vi "selectDailySummary.vi"(8 "Shift":string="中", 10 "End_date":string="2014/11/13", 11 "Begin_date":string="2014/11/12") -> (2 "Summary":string[][](array[string]))   [LabVIEW 2012]
uses:
  <vilib>/addons/database/Auxilliary.llb/DB Tools Cursor Type.ctl
  <vilib>/addons/database/Connection.llb/DB Tools Open Connec (Path).vi
  <vilib>/addons/database/Connection.llb/Conn Execute.vi
  <vilib>/addons/database/Recordset.llb/Rec Fetch Recordset Data (R).vi
  <vilib>/addons/database/Recordset.llb/Rec Destroy - Connection.vi
  <vilib>/addons/database/_DB Variant To Data/Database Variant To Data.xnode
  <vilib>/addons/database/NI_Database_API.lvlib
panel:
  out "concatenated string":string
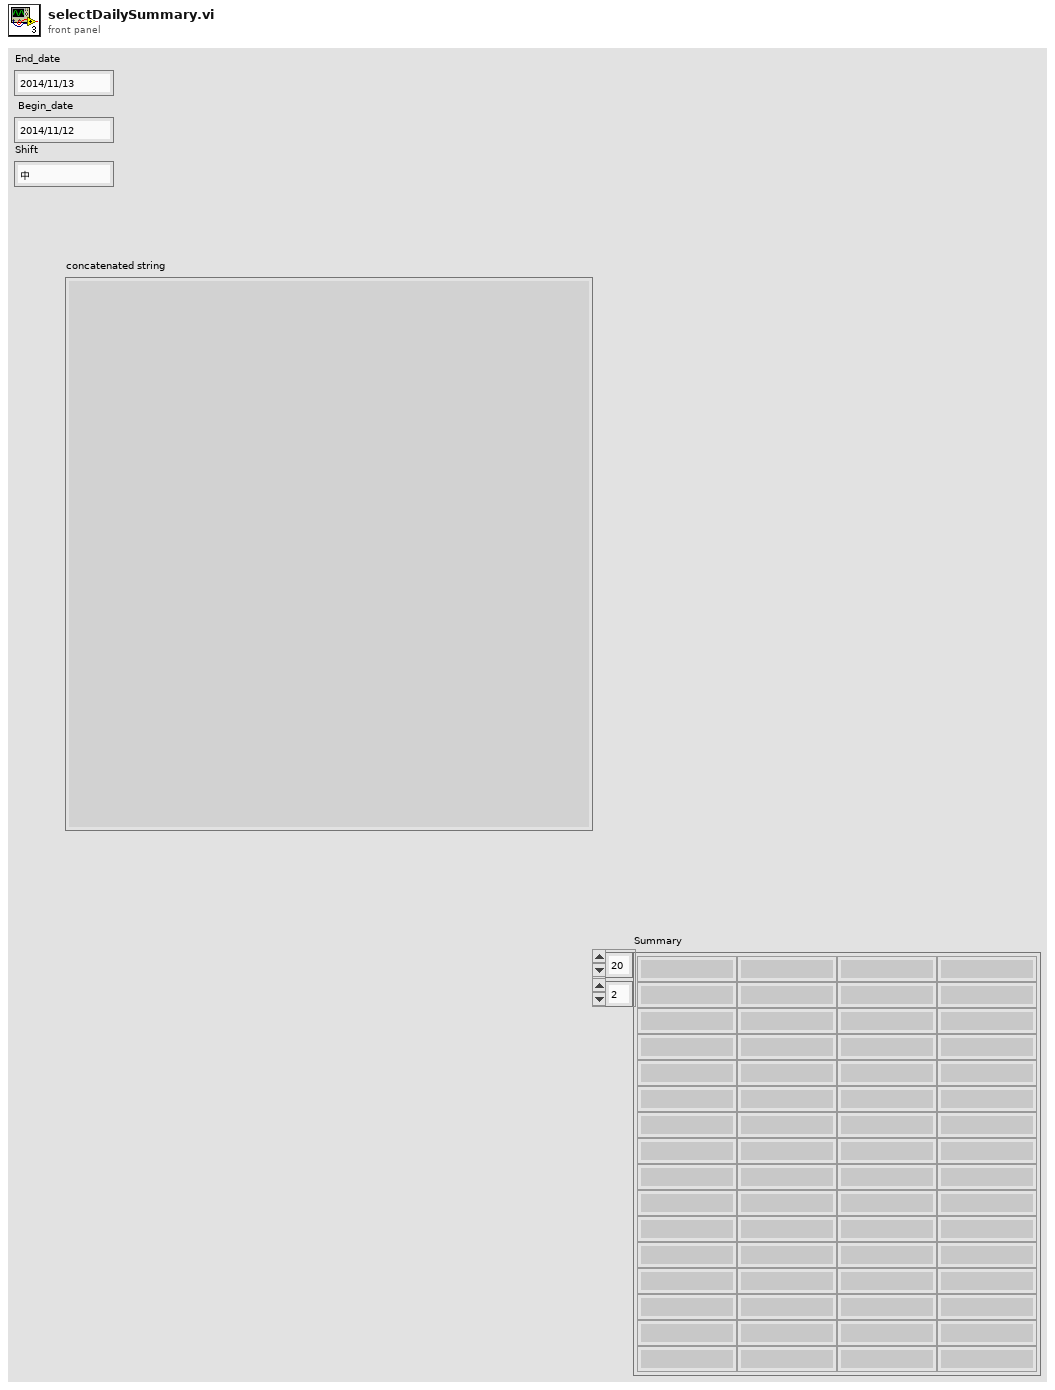
[diagram p1: front panel]
types:
  T1 = typedef "NI_Database_API.lvlib/DB Tools Cursor Type.ctl" = enum16{"forward-only", "keyset", "dynamic", "static"}
  T2 = typedef "NI_Database_API.lvlib/Conn ObjectReference.ctl" = refnum<k1>
  T3 = typedef "NI_Database_API.lvlib/Rec ObjectReference.ctl" = refnum<k1>
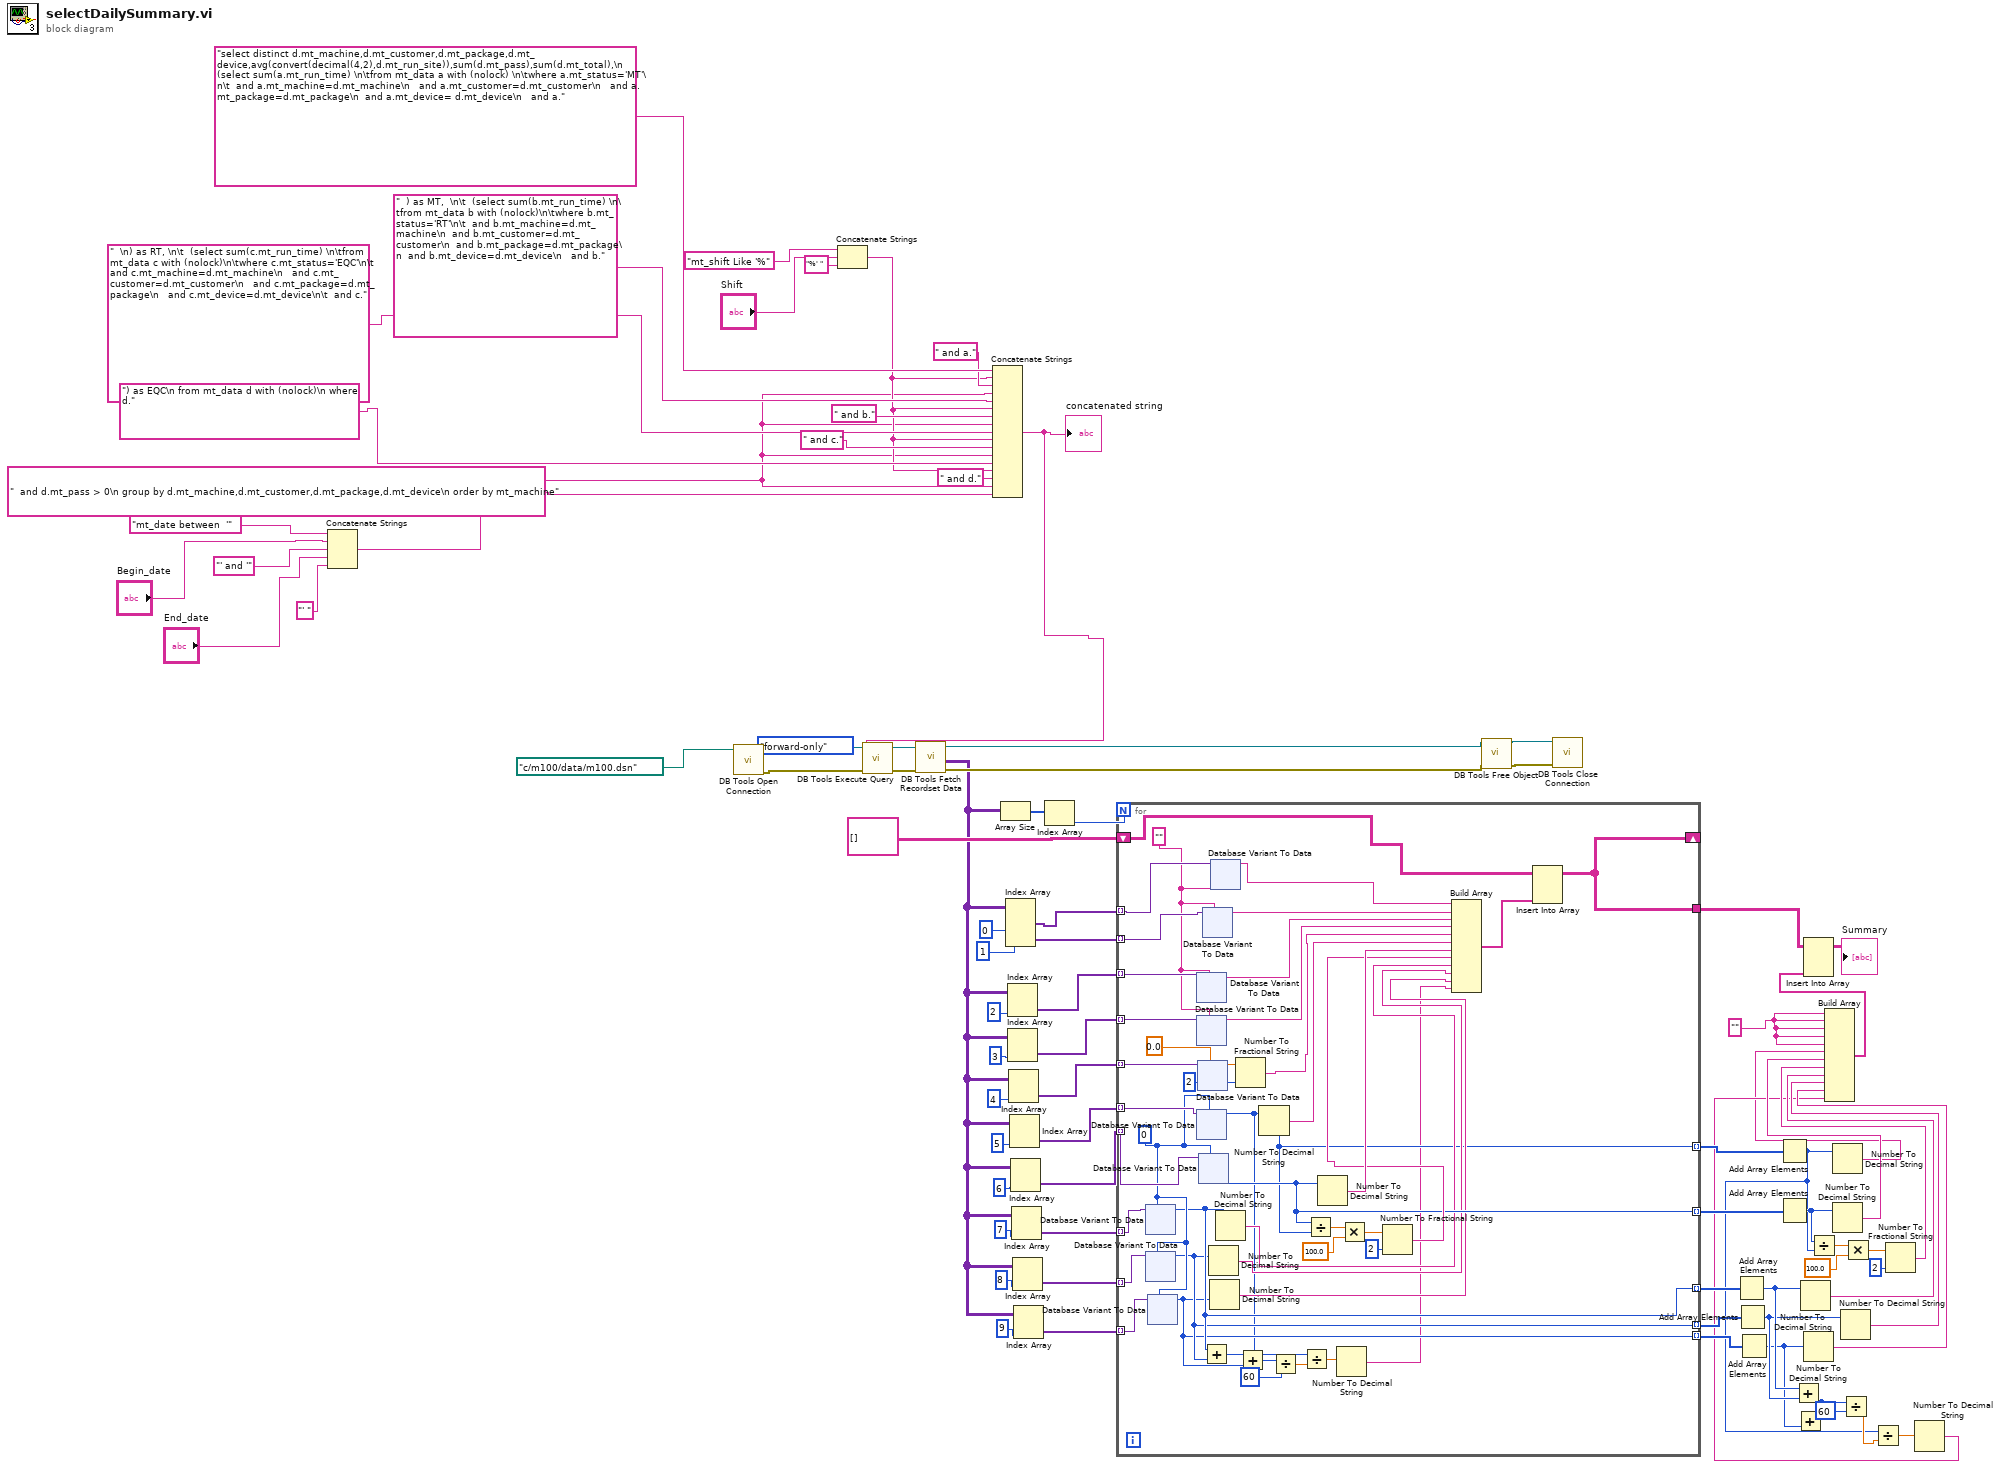
[diagram p0: block diagram]
diagram:
  w1 = "" ("element")
  n1 = Concatenate Strings("mt_date between  '", "Begin_date", "' and '" ("string"), "End_date", "' " ("string")) -> (w10:string)
  n2 = call-poly <vilib>:"DB Tools Open Connection.vi"("connection information"=path "c:/m100/data/m100.dsn") -> ("error out"=w56:errorcluster, "connection reference"=w57:T2)  [unwired: 7 in]
  n3 = Concatenate Strings("mt_shift Like '%" ("string"), "Shift", "%' " ("string")) -> (w12:string)
  n4 = Concatenate Strings("select distinct d.mt_machine,d.mt_customer,d.mt_package,d.mt_device,avg(convert(decimal(4,2),d.mt_run_site)),sum(d.mt_pass),sum(d.mt_total),\n (select sum(a.mt_run_time) \n\tfrom mt_data a with (nolock) \n\twhere a.mt_status='MT'\n\t  and a.mt_machine=d.mt_machine\n   and a.mt_customer=d.mt_customer\n   and a.mt_package=d.mt_package\n  and a.mt_device= d.mt_device\n   and a." ("string"), w12, " and a." ("string"), w10, "  ) as MT,  \n\t  (select sum(b.mt_run_time) \n\tfrom mt_data b with (nolock)\n\twhere b.mt_status='RT'\n\t  and b.mt_machine=d.mt_machine\n  and b.mt_customer=d.mt_customer\n  and b.mt_package=d.mt_package\n  and b.mt_device=d.mt_device\n   and b." ("string"), w12, " and b." ("string"), w10, "  \n) as RT, \n\t  (select sum(c.mt_run_time) \n\tfrom mt_data c with (nolock)\n\twhere c.mt_status='EQC'\n\t  and c.mt_machine=d.mt_machine\n   and c.mt_customer=d.mt_customer\n   and c.mt_package=d.mt_package\n   and c.mt_device=d.mt_device\n\t  and c." ("string"), w12, " and c." ("string"), w10, ") as EQC\n from mt_data d with (nolock)\n where d." ("string"), w12, " and d." ("string"), w10, "  and d.mt_pass > 0\n group by d.mt_machine,d.mt_customer,d.mt_package,d.mt_device\n order by mt_machine" ("string")) -> (w7:string)
  "concatenated string" <- w7
  n5 = call-poly <vilib>:"DB Tools Execute Query.vi"("error in (no error)"=w56, "cursor type"=DB_Tools_Cursor_Type."forward-only", "SQL query"=w7, "connection reference"=w57) -> ("error out"=w59:errorcluster, "recordset reference"=w58:T3)  [unwired: 4 in]
  n6 = call-poly <vilib>:"DB Tools Fetch Recordset Data.vi"("error in (no error)"=w59, "recordset reference"=w58) -> ("error out"=w55:errorcluster, "recordset data"=w6:variant[][], "recordset reference out"=w54:T3)  [unwired: 3 in]
  n7 = Array Size(array=w6) -> (size(s)=w83:i32[])
  n8 = Index Array(array=w6, index (col) #1=0 ("disabled index (col)"), index (col) #2=1 ("index (col)")) -> (element #1=w4:variant[], element #2=w2:variant[])  [unwired: 2 in]
  n9 = Index Array(array=w6, index (col)=2) -> (element=w76:variant[])  [unwired: 1 in]
  n10 = Index Array(array=w6, index (col)=3) -> (element=w75:variant[])  [unwired: 1 in]
  n11 = Index Array(array=w6, index (col)=4) -> (element=w71:variant[])  [unwired: 1 in]
  n12 = Index Array(array=w6, index (col)=5) -> (element=w74:variant[])  [unwired: 1 in]
  n13 = Index Array(array=w6, index (col)=6) -> (element=w73:variant[])  [unwired: 1 in]
  n14 = Index Array(array=w6, index (col)=7) -> (element=w48:variant[])  [unwired: 1 in]
  n15 = Index Array(array=w6, index (col)=8) -> (element=w47:variant[])  [unwired: 1 in]
  n16 = Index Array(array=w6, index (col)=9) -> (element=w46:variant[])  [unwired: 1 in]
  n17 = Index Array(array=w83) -> (element=w82:i32)  [unwired: 1 in]
  n18 = for {
    N: w82 -> [_]
    tunnel: w73 -> [w127] mode=indexing
    shift-right: [w110] -> _
    shift-left: string[][] [] -> [w113]
    tunnel: w76 -> [w126] mode=indexing
    tunnel: w75 -> [w125] mode=indexing
    tunnel: w74 -> [w124] mode=indexing
    tunnel: w71 -> [w121] mode=indexing
    tunnel: [w95] -> w36 mode=indexing
    tunnel: [w115] -> w70 mode=indexing
    tunnel: [w110] -> w52
    tunnel: w48 -> [w109] mode=indexing
    tunnel: w47 -> [w108] mode=indexing
    tunnel: w46 -> [w107] mode=indexing
    tunnel: [w99] -> w43 mode=indexing
    tunnel: [w101] -> w44 mode=indexing
    tunnel: [w102] -> w45 mode=indexing
    tunnel: w4 -> [w92] mode=indexing
    tunnel: w2 -> [w91] mode=indexing
    w106 = 0
    w90 = ""
    n19 = xnode "Database Variant To Data"("database variant"=w109, "type"=w106) -> ("data"=w102:i32)  [unwired: 1 in, 1 out]
    n20 = xnode "Database Variant To Data"("database variant"=w108, "type"=w106) -> ("data"=w101:i32)  [unwired: 1 in, 1 out]
    n21 = xnode "Database Variant To Data"("database variant"=w107, "type"=w106) -> ("data"=w99:i32)  [unwired: 1 in, 1 out]
    n22 = xnode "Database Variant To Data"("database variant"=w126, "type"=w90) -> ("data"=w112:string)  [unwired: 1 in, 1 out]
    n23 = xnode "Database Variant To Data"("database variant"=w125, "type"=w90) -> ("data"=w111:string)  [unwired: 1 in, 1 out]
    n24 = xnode "Database Variant To Data"("database variant"=w124, "type"=w106) -> ("data"=w95:i32)  [unwired: 1 in, 1 out]
    n25 = xnode "Database Variant To Data"("database variant"=w121, "type"=0.0) -> ("data"=w86:dbl)  [unwired: 1 in, 1 out]
    n26 = xnode "Database Variant To Data"("database variant"=w127, "type"=w106) -> ("data"=w115:i32)  [unwired: 1 in, 1 out]
    n27 = Add(x=w102, y=w101) -> (x+y=w100:i32)
    n28 = xnode "Database Variant To Data"("database variant"=w91, "type"=w90) -> ("data"=w88:string)  [unwired: 1 in, 1 out]
    n29 = Number To Decimal String(number=w101) -> (decimal integer string=w104:string)  [unwired: 1 in]
    n30 = Number To Decimal String(number=w99) -> (decimal integer string=w103:string)  [unwired: 1 in]
    n31 = xnode "Database Variant To Data"("database variant"=w92, "type"=w90) -> ("data"=w89:string)  [unwired: 1 in, 1 out]
    n32 = Number To Decimal String(number=w102) -> (decimal integer string=w105:string)  [unwired: 1 in]
    n33 = Number To Fractional String(number=w86, precision (6)=i16 2) -> (F-format string=w85:string)  [unwired: 2 in]
    n34 = Add(x=w100, y=w99) -> (x+y=w98:i32)
    n35 = Number To Decimal String(number=w95) -> (decimal integer string=w119:string)  [unwired: 1 in]
    n36 = Divide(x=w98, y=60) -> (x/y=w96:dbl)
    n37 = Divide(x=w95, y=w96) -> (x/y=w94:dbl)
    n38 = Divide(x=w115, y=w95) -> (x/y=w122:dbl)
    n39 = Number To Decimal String(number=w115) -> (decimal integer string=w120:string)  [unwired: 1 in]
    n40 = Number To Decimal String(number=w94) -> (decimal integer string=w93:string)  [unwired: 1 in]
    n41 = Multiply(x=w122, y=100.0) -> (x*y=w118:dbl)
    n42 = Number To Fractional String(number=w118, precision (6)=i16 2) -> (F-format string=w117:string)  [unwired: 2 in]
    n43 = Build Array(w89, w88, w112, w111, w85, w119, w120, w117, w105, w104, w103, w93) -> (w114:string[])
    n44 = Insert Into Array(array=w113, new element=w114) -> (w110:string[][])  [unwired: 2 in]
  }
  n45 = call-poly <vilib>:"DB Tools Free Object.vi"("error in (no error)"=w55, "recordset reference"=w54) -> ("error out"=w60:errorcluster, "connection reference"=w61:T2)  [unwired: 8 in]
  n46 = call <vilib>:"DB Tools Close Connection.vi"("error in (no error)"=w60, "connection reference"=w61) -> ()  [unwired: 5 in, 1 out]
  n47 = Add Array Elements(numeric array=w45) -> (sum=w39:i32)
  n48 = Add Array Elements(numeric array=w44) -> (sum=w38:i32)
  n49 = Add Array Elements(numeric array=w43) -> (sum=w37:i32)
  n50 = Add Array Elements(numeric array=w36) -> (sum=w30:i32)
  n51 = Add Array Elements(numeric array=w70) -> (sum=w63:i32)
  n52 = Add(x=w39, y=w38) -> (x+y=w35:i32)
  n53 = Add(x=w35, y=w37) -> ()  [unwired: 1 out]
  n54 = Number To Decimal String(number=w39) -> (decimal integer string=w42:string)  [unwired: 1 in]
  n55 = Number To Decimal String(number=w37) -> (decimal integer string=w40:string)  [unwired: 1 in]
  n56 = Divide(x=w63, y=w30) -> (x/y=w66:dbl)
  n57 = Number To Decimal String(number=w30) -> (decimal integer string=w29:string)  [unwired: 1 in]
  n58 = Number To Decimal String(number=w63) -> (decimal integer string=w69:string)  [unwired: 1 in]
  n59 = Number To Decimal String(number=w38) -> (decimal integer string=w41:string)  [unwired: 1 in]
  n60 = Divide(x=w35, y=60) -> (x/y=w33:dbl)
  n61 = Multiply(x=w66, y=100.0) -> (x*y=w65:dbl)
  n62 = Divide(x=w30, y=w33) -> (x/y=w32:dbl)
  n63 = Number To Fractional String(number=w65, precision (6)=i16 2) -> (F-format string=w62:string)  [unwired: 2 in]
  n64 = Number To Decimal String(number=w32) -> (decimal integer string=w31:string)  [unwired: 1 in]
  n65 = Build Array(w1, w1, w1, w1, w1, w29, w69, w62, w42, w41, w40, w31) -> (w68:string[])
  n66 = Insert Into Array(array=w52, new element=w68) -> (→"Summary":string[][])  [unwired: 2 in]
